vi "Test App Get Process Before Starting App.vi"(8 "error in (no error)":errorcluster, 11 "Rig Test in":refnum<class "Application Dev Test.lvclass">) -> (0 "error out":errorcluster, 3 "Rig Test out":refnum<class "Application Dev Test.lvclass">)   [LabVIEW 2020, in "Application Dev Test.lvclass"]
uses:
  Application Dev Test.lvclass
  C:/Program Files (x86)/National Instruments/LabVIEW 2020/vi.lib/Astemes/LUnit/Test Case.lvclass
  source/Framework/Process/Process.lvclass
  source/Framework/Process/Process.lvclass/Process.ctl
  source/Framework/Application/Application.lvclass/Application.ctl
  <vilib>/Astemes/LUnit/Test Case.lvclass/Test Case.ctl
  source/Framework/Application/Private/Add Process to Map.vi
  source/Framework/Application/Private/Throw Error If Process Already in App.vi
  source/Framework/Process/Protected/Messaging/Send Message.vi
  source/Framework/Process/Public/Lifecycle/Get Lifecycle State.vi
  source/Framework/Process/Protected/SubVIs/Set Context.vi
  source/Framework/Application/Private/Retrieve Process from App.vi
  source/Framework/Application/Private/Parse Process Name.vi
  source/Framework/Application/Private/Get Process from Map.vi
  <vilib>/Astemes/LUnit/Palette/Fail.vi
  <vilib>/Astemes/LUnit/Palette/Pass.vi
  <vilib>/Astemes/LUnit/Set Assertion Type.vi
  source/Framework/Process/Private/SubVIs/Handle Debug Data.vi
  <vilib>/Utility/error.llb/Clear Errors.vi
  source/Framework/Process/Public/Lifecycle/Leave Process Loop.vi
  source/Framework/Process/Protected/Messaging/Request Message.vi
  <vilib>/AdvancedString/Delimited String to 1D String Array.vi
  <vilib>/Astemes/LUnit/Add test result.vi
  source/Framework/Logging/Log Debug.vi
  <vilib>/AdvancedString/1D String Array to Delimited String.vi
  <vilib>/Utility/High Resolution Relative Seconds.vi
  source/Framework/Process/Private/SubVIs/Enqueue Request Message.vi
  <vilib>/Astemes/LUnit/LUnit Record Assertion Result.vi
  <vilib>/Astemes/LUnit/LUnit Aggregate Assertion Results.vi
  <vilib>/Astemes/LUnit/Method Result/LUnit Merge Status.vi
  <vilib>/Astemes/LUnit/LUnit Concatenate result strings.vi
  source/Framework/Application/Application.lvclass
  C:/Git/astemes-triarc-framework/source/Framework/Process/Process.lvclass
  <vilib>/Utility/error.llb/Error Cluster From Error Code.vi
  source/Framework/Process/Public/Read Name.vi
  source/Framework/Process/Private/SubVIs/Wait for Response Message.vi
  <vilib>/Astemes/LUnit/Test Case.lvclass
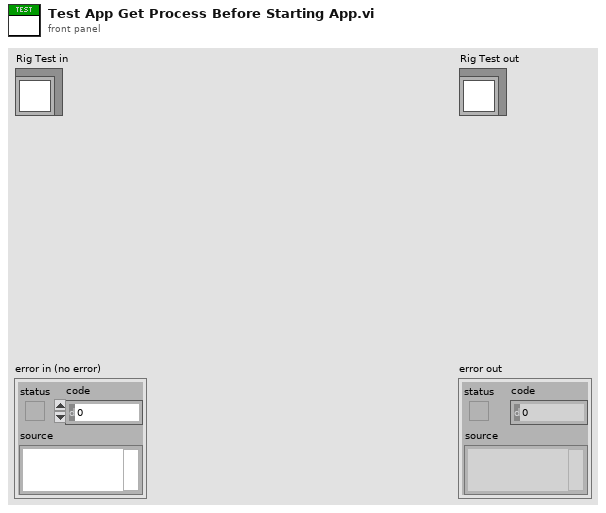
[diagram p1: front panel]
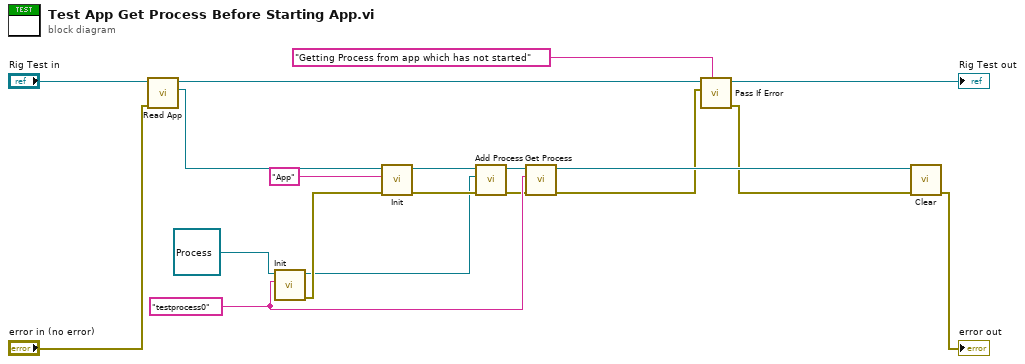
[diagram p0: block diagram]
diagram:
  w11 = "testprocess0" ("Name")
  n1 = call "Read App.vi"("error in (no error)"="error in (no error)", "Application Test In"="Rig Test in") -> ("App out"=w18:refnum<class "Application.lvclass">, "Application Test Out"=w10:refnum<class "Application Dev Test.lvclass">)  [unwired: 7 in, 1 out]
  n2 = call-dynamic "Init.vi"("Name"=w11, "Process In"=refnum<class "Process.lvclass"> refnum ("Process.lvclass")) -> ("error out"=w6:errorcluster, "Process Out"=w3:refnum<class "Process.lvclass">)  [unwired: 8 in]
  n3 = call-dynamic "Init.vi"("error in (no error)"=w6, "Name"="App", "Process In"=w18) -> ("error out"=w13:errorcluster, "Process Out"=w15:refnum<class "Application.lvclass">)  [unwired: 7 in]
  n4 = call "Add Process.vi"("error in (no error)"=w13, "Process"=w3, "Application In"=w15) -> ("error out"=w2:errorcluster, "Application Out"=w16:refnum<class "Application.lvclass">)  [unwired: 7 in]
  n5 = call "Get Process.vi"("error in (no error)"=w2, "Process Name"=w11, "Application In"=w16) -> ("error out"=w1:errorcluster, "Application Out"=w14:refnum<class "Application.lvclass">)  [unwired: 6 in, 1 out]
  n6 = call <vilib>:"Pass If Error.vi"("Description"="Getting Process from app which has not started", "Assert error"=w1, "LUnit Test Case In"=w10) -> ("error out"=w7:errorcluster, "LUnit Test Case Out"=→"Rig Test out":refnum<class "Application Dev Test.lvclass">)  [unwired: 7 in]
  n7 = call-dynamic "Clear.vi"("error in (no error)"=w7, "Application In"=w14) -> ("error out"=→"error out":errorcluster)  [unwired: 9 in]
